vi "Disable_Children.vi"(8 "error in (no error)":errorcluster, 10 "Tree item":refnum<class "IB_Tree_Item.lvclass">, 11 "IB_Tree in":refnum<class "IB_Tree.lvclass">) -> (0 "error out":errorcluster, 3 "IB_Tree out":refnum<class "IB_Tree.lvclass">)   [LabVIEW 2020, in "IB_Tree.lvclass"]
uses:
  <vilib>/AppBuilder/IB_Classes/Tree/IB_Tree.lvclass
  <vilib>/AppBuilder/IB_Classes/Tree/IB_Tree.lvclass/IB_Tree.ctl
  <vilib>/AppBuilder/IB_Classes/Tree_Item/IB_Tree_Item.lvclass
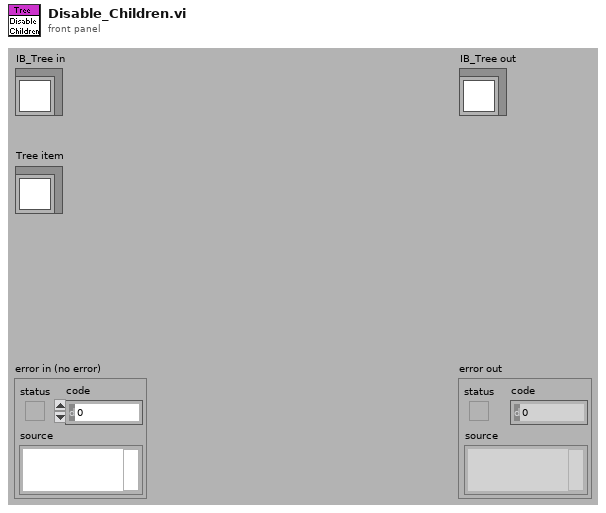
[diagram p1: front panel]
types:
  T1 = typedef "IB_Tree_Item.ctl" = cluster{"symbol index":i32, "child tag":string, "parentTag":string, "left cell name":string}
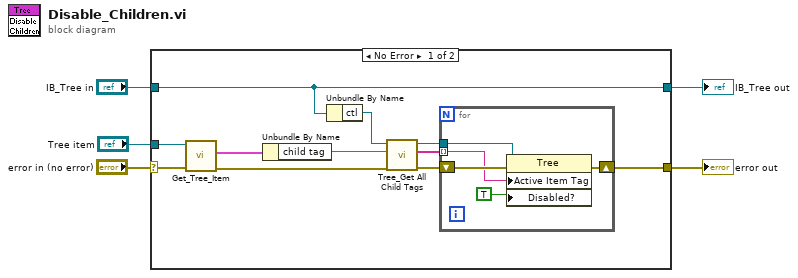
[diagram p0: block diagram]
diagram:
  n1 = case shown="No Error" "error in (no error)" {
    selector: "error in (no error)" -> [w7 w23]
    tunnel: [w11 w23] -> w4
    tunnel: [w16 w22] -> w2
    tunnel: "IB_Tree in" -> [w16 w22]
    tunnel: "Tree item" -> [w10 _]
    frame No Error {
      n2 = call <vilib>:"Get_Tree_Item.vi"("error in (no error)"=w7, "IB_TreeItem in"=w10) -> ("error out"=w6:errorcluster, "data"=w9:T1)  [unwired: 7 in, 1 out]
      n3 = Unbundle By Name(w9) -> ("child tag"=w8:string)
      n4 = Unbundle By Name(w16) -> ("ctl"=w15:refnum<vi>)
      n5 = call <vilib>:"Tree_Get All Child Tags.vi"("error in (no error)"=w6, "Parent Tag"=w8, "Tree Refnum"=w15) -> ("error out"=w12:errorcluster, "All Child Tags"=w14:string[], "dup Tree Refnum"=w13:refnum<vi>)  [unwired: 6 in]
      n6 = for {
        tunnel: w14 -> [w19] mode=indexing
        tunnel: w13 -> [w21]
        shift-right: [w18] -> w11
        shift-left: w12 -> [w20]
        n7 = property class="Tree"(reference=w21, error in=w20, "Active Item Tag"=w19, "Disabled?"=TRUE ("Active Item:Disabled?")) -> (error out=w18:errorcluster)  [unwired: 1 out]
      }
    }
    frame Error {
    }
  }
  "error out" <- w4
  "IB_Tree out" <- w2
